vi "Calibration and Function folders.vi"(11 "Folder":T1) -> (7 "Selected Folder":path)   [LabVIEW 2015]
uses:
  DAC project/Calibration and Function folders.ctl
  <vilib>/Utility/sysdir.llb/System Directory Type.ctl
panel:
  out "appended path":path
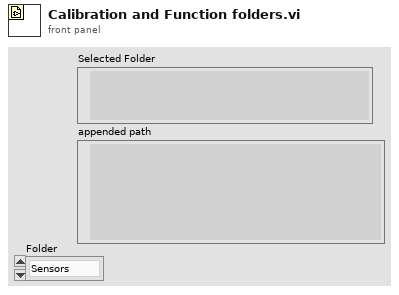
[diagram p1: front panel]
types:
  T1 = typedef "Calibration and Function folders.ctl" = enum16{"Sensors", "Functions", "Config File", "UserAppFolder"}
  T2 = enum16{"open", "replace", "create", "open or create", "replace or create", "replace or create with confirmation"}
  T3 = typedef "System Directory Type.ctl" = i32
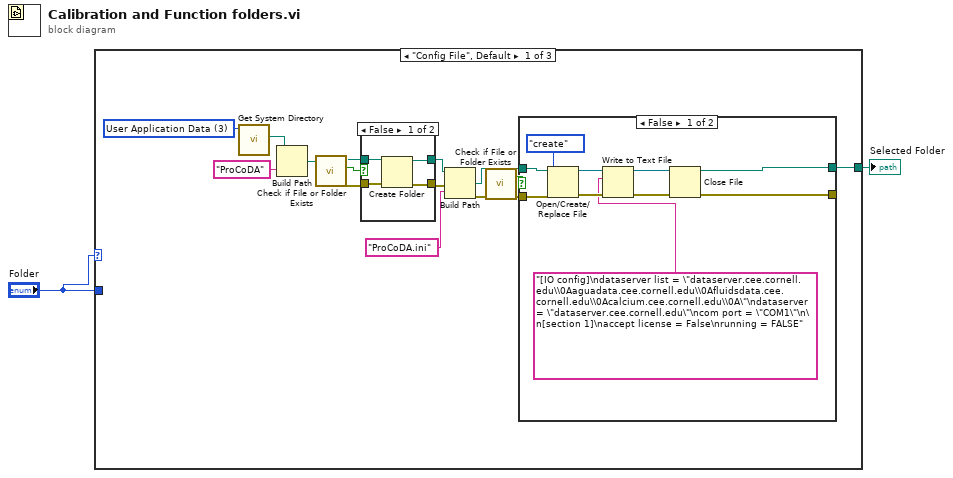
[diagram p0: block diagram]
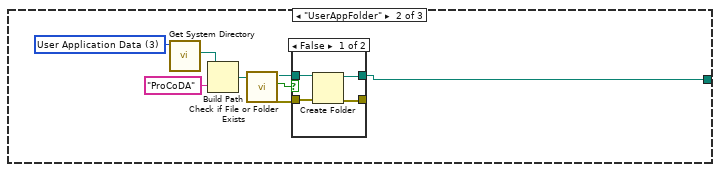
[diagram p4: hidden frame]
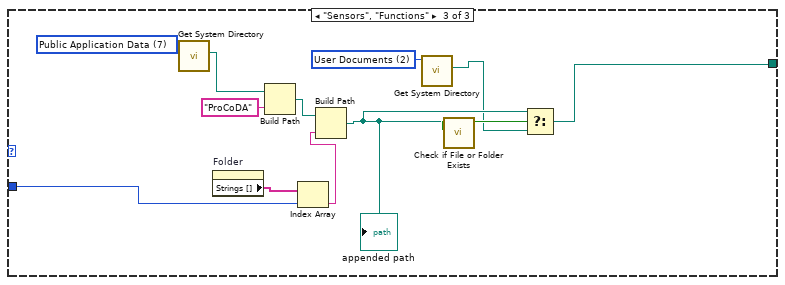
[diagram p6: hidden frame]
diagram:
  n1 = case shown="\"Config File\", Default" "Folder" {
    tunnel: [w3 w36 w56] -> w2
    tunnel: "Folder" -> [_ _ w54]
    frame "Config File", Default {
      w17 = T3 3 items=["User Home"=0, "User Desktop"=1, "User Documents"=2, "User Application Data"=3, "User Preferences"=4, "User Temporary"=5, "Public Documents"=6, "Public Application Data"=7, "Public Preferences"=8, "Public Cache"=13, "System Core Libraries"=9, "System Installed Libraries"=10, "Application Files"=11, "Boot Volume Root"=12] ("system directory type")
      n2 = call <vilib>:"Get System Directory.vi"("system directory type"=w17) -> ("system directory"=w15:path)  [unwired: 10 in]
      n3 = Build Path(base path=w15, name or relative path="ProCoDA") -> (appended path=w14:path)
      n4 = call <vilib>:"Check if File or Folder Exists.vi"("path"=w14) -> ("error out"=w11:errorcluster, "file or folder exists?"=w13:bool, "dup path"=w12:path)  [unwired: 8 in]
      n5 = case shown="False" w13 {
        tunnel: w12 -> [w33 w35]
        tunnel: w11 -> [w32 w34]
        tunnel: [w31 w35] -> w9
        tunnel: [w30 w34] -> w7
        frame False {
          n6 = Create Folder(path (use dialog)=w33, error in=w32) -> (created path=w31:path, error out=w30:errorcluster)  [unwired: 1 in, 1 out]
        }
        frame True {
        }
      }
      n7 = Build Path(base path=w9, name or relative path="ProCoDA.ini") -> (appended path=w8:path)
      n8 = call <vilib>:"Check if File or Folder Exists.vi"("error in (no error)"=w7, "path"=w8) -> ("error out"=w5:errorcluster, "file or folder exists?"=w6:bool, "dup path"=w4:path)  [unwired: 7 in]
      n9 = case shown="False" w6 {
        tunnel: w5 -> [w27 w28]
        tunnel: w4 -> [w26 w29]
        tunnel: [w24 w29] -> w3
        tunnel: [w23 w28] -> _
        frame False {
          n10 = Open/Create/Replace File(file path (use dialog)=w26, error in=w27, operation (0:open)=T2."create") -> (refnum out=w20:refnum<file>, error out=w22:errorcluster)  [unwired: 3 in, 1 out]
          n11 = Write to Text File(file (use dialog)=w20, text="[IO config]\ndataserver list = \"dataserver.cee.cornell.edu\\0Aaguadata.cee.cornell.edu\\0Afluidsdata.cee.cornell.edu\\0Acalcium.cee.cornell.edu\\0A\"\ndataserver = \"dataserver.cee.cornell.edu\"\ncom port = \"COM1\"\n\n[section 1]\naccept license = False\nrunning = FALSE", error in=w22) -> (refnum out=w19:refnum<file>, error out=w21:errorcluster)  [unwired: 1 in, 1 out]
          n12 = Close File(refnum=w19, error in=w21) -> (path=w24:path, error out=w23:errorcluster)
        }
        frame True {
        }
      }
    }
    frame "UserAppFolder" {
      w43 = T3 3 items=["User Home"=0, "User Desktop"=1, "User Documents"=2, "User Application Data"=3, "User Preferences"=4, "User Temporary"=5, "Public Documents"=6, "Public Application Data"=7, "Public Preferences"=8, "Public Cache"=13, "System Core Libraries"=9, "System Installed Libraries"=10, "Application Files"=11, "Boot Volume Root"=12] ("system directory type")
      n13 = call <vilib>:"Get System Directory.vi"("system directory type"=w43) -> ("system directory"=w41:path)  [unwired: 10 in]
      n14 = Build Path(base path=w41, name or relative path="ProCoDA") -> (appended path=w40:path)
      n15 = call <vilib>:"Check if File or Folder Exists.vi"("path"=w40) -> ("error out"=w37:errorcluster, "file or folder exists?"=w39:bool, "dup path"=w38:path)  [unwired: 8 in]
      n16 = case shown="False" w39 {
        tunnel: w38 -> [w47 w49]
        tunnel: w37 -> [w46 w48]
        tunnel: [w45 w49] -> w36
        tunnel: [w44 w48] -> _
        frame False {
          n17 = Create Folder(path (use dialog)=w47, error in=w46) -> (created path=w45:path, error out=w44:errorcluster)  [unwired: 1 in, 1 out]
        }
        frame True {
        }
      }
    }
    frame "Sensors", "Functions" {
      w52 = T3 2 items=["User Home"=0, "User Desktop"=1, "User Documents"=2, "User Application Data"=3, "User Preferences"=4, "User Temporary"=5, "Public Documents"=6, "Public Application Data"=7, "Public Preferences"=8, "Public Cache"=13, "System Core Libraries"=9, "System Installed Libraries"=10, "Application Files"=11, "Boot Volume Root"=12] ("system directory type")
      w61 = T3 7 items=["User Home"=0, "User Desktop"=1, "User Documents"=2, "User Application Data"=3, "User Preferences"=4, "User Temporary"=5, "Public Documents"=6, "Public Application Data"=7, "Public Preferences"=8, "Public Cache"=13, "System Core Libraries"=9, "System Installed Libraries"=10, "Application Files"=11, "Boot Volume Root"=12] ("system directory type")
      n18 = call <vilib>:"Get System Directory.vi"("system directory type"=w61) -> ("system directory"=w51:path)  [unwired: 10 in]
      n19 = property on="Folder" class="Enum (strict)"() -> ("Strings []"=w55:string[])  [unwired: 2 in, 2 out]
      n20 = Build Path(base path=w51, name or relative path="ProCoDA") -> (appended path=w59:path)
      n21 = Index Array(array=w55, index=w54) -> (element=w53:string)
      n22 = Build Path(base path=w59, name or relative path=w53) -> (appended path=w57:path)
      "appended path" <- w57
      n23 = call <vilib>:"Get System Directory.vi"("system directory type"=w52) -> ("system directory"=w50:path)  [unwired: 10 in]
      n24 = call <vilib>:"Check if File or Folder Exists.vi"("path"=w57) -> ("file or folder exists?"=w58:bool)  [unwired: 8 in, 2 out]
      n25 = Select(t=w57, s=w58, f=w50) -> (s? t:f=w56:path)
    }
  }
  "Selected Folder" <- w2
